vi "Close.vi"(8 "error in (no error)":errorcluster caption="entrée d'erreur (pas d'erreur)", 11 "Class Printer_CAB en entrée":refnum<class "Class Printer_TSC.lvclass">) -> (0 "error out":errorcluster caption="sortie d'erreur", 3 "Class Printer_CAB en sortie":refnum<class "Class Printer_TSC.lvclass">)   [LabVIEW 2020, in "Library Instrument & Equipement.lvlib" / "Library Printer.lvlib" / "Class Printer_TSC.lvclass"]
uses:
  Class Printer_TSC.lvclass
  Printer (Default)/Class Printer (Default).lvclass
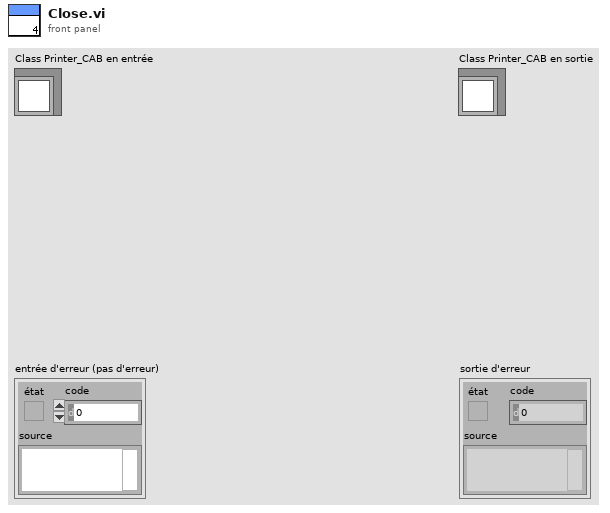
[diagram p1: front panel]
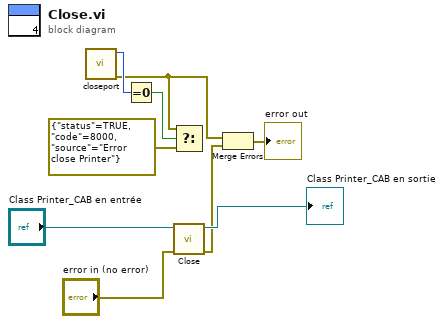
[diagram p0: block diagram]
diagram:
  n1 = call "closeport.vi"() -> ("error out"=w1:errorcluster, "function return"=w3:i32)  [unwired: 10 in]
  n2 = Equal To 0?(x=w3) -> (x = 0?=w4:bool)
  n3 = Select(t=w1, s=w4, f=errorcluster {"status"=TRUE, "code"=8000, "source"="Error close Printer"} ("cas vrai")) -> ()  [unwired: 1 out]
  n4 = call-parent "Close.vi"("error in (no error)"="error in (no error)", "Class Printer (Default) en entrée"="Class Printer_CAB en entrée") -> ("error out"=w6:errorcluster, "Class Printer (Default) en sortie"=→"Class Printer_CAB en sortie":refnum<class "Class Printer_TSC.lvclass">)  [unwired: 8 in]
  n5 = Merge Errors(w1, w6) -> (→"error out":errorcluster)
